vi "Trajectory_RelativeTo.vi"(9 "POSE":T3={"TRANSLATION"={"X"=0.0, "Y"=0.0}, "ROTATION"={"VALUE"=0.0, "COS"=1.0, "SIN"=0.0}} {"ROTATION"."SIN" format="%13.4f"; "ROTATION"."COS" format="%13.4f"; "ROTATION"."VALUE" format="%13.4f"; "TRANSLATION"."Y" format="%14.3f"; "TRANSLATION"."X" format="%14.3f"}, 11 "InputTRAJECTORY":T1 {"States"."POSE"."ROTATION"."SIN" format="%13.4f"; "States"."POSE"."ROTATION"."COS" format="%13.4f"; "States"."POSE"."ROTATION"."VALUE" format="%13.4f"; "States"."POSE"."TRANSLATION"."Y" format="%14.3f"; "States"."POSE"."TRANSLATION"."X" format="%14.3f"; "TotalTImeSecs" format="%20.3f"}) -> (3 "outputTRAJECTORY":T1 {"States"."POSE"."ROTATION"."SIN" format="%13.4f"; "States"."POSE"."ROTATION"."COS" format="%13.4f"; "States"."POSE"."ROTATION"."VALUE" format="%13.4f"; "States"."POSE"."TRANSLATION"."Y" format="%14.3f"; "States"."POSE"."TRANSLATION"."X" format="%14.3f"; "TotalTImeSecs" format="%20.3f"})   [LabVIEW 2019, in "Trajectory_Library.lvlib"]
doc: "Transforms all poses in the trajectory so that they are relative to the given pose. This is useful for converting a field-relative trajectory into a robot-relative trajectory.\n \nParameters:\n - InputTrajectory - Trajectory data structure\n - pose -The pose that is the origin of the coordinate frame that the current trajectory will be transformed into.\n \nReturns:\n - OutputTrajectory - The transformed trajectory."
uses:
  Trajectory_Library.lvlib
  TypeDef/TRANSLATION2D.ctl
  TypeDef/ROTATION2D.ctl
  TypeDef/POSE2D.ctl
  TypeDef/TRAJ_STATE.ctl
  TypeDef/TRAJECTORY.ctl
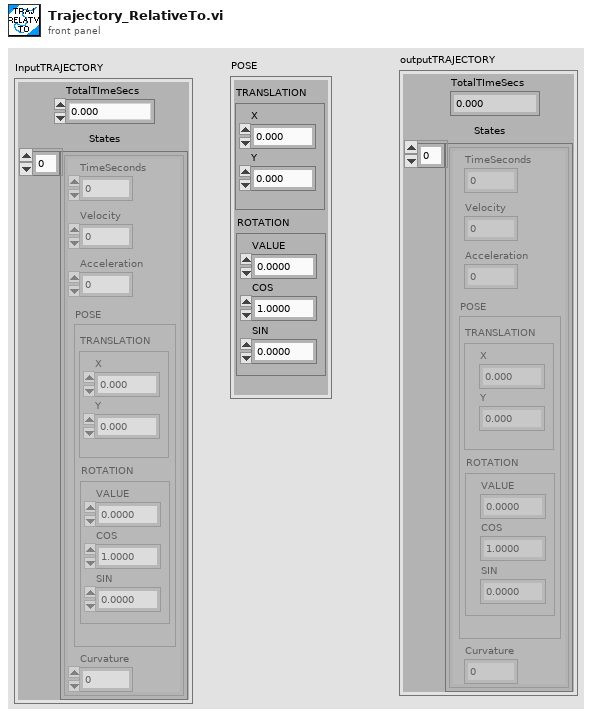
[diagram p1: front panel]
types:
  T1 = typedef "Trajectory_Library.lvlib/TRAJECTORY.ctl" = cluster{"TotalTImeSecs":dbl, "States":T2[]}
  T2 = typedef "Trajectory_Library.lvlib/TRAJ_STATE.ctl" = cluster{"TimeSeconds":dbl, "Velocity":dbl, "Acceleration":dbl, "POSE":T3, "Curvature":dbl}
  T3 = typedef "Trajectory_Library.lvlib/POSE2D.ctl" = cluster{"TRANSLATION":T4, "ROTATION":T5}
  T4 = typedef "Trajectory_Library.lvlib/TRANSLATION2D.ctl" = cluster{"X":dbl, "Y":dbl}
  T5 = typedef "Trajectory_Library.lvlib/ROTATION2D.ctl" = cluster{"VALUE":dbl, "COS":dbl, "SIN":dbl}
  T6 = typedef "WPILib_Math.lvlib/TRAJ_STATE.ctl" = cluster{"TimeSeconds":dbl, "Velocity":dbl, "Acceleration":dbl, "POSE":T7, "Curvature":dbl}
  T7 = typedef "WPILib_Math.lvlib/POSE2D.ctl" = cluster{"TRANSLATION":T8, "ROTATION":T9}
  T8 = typedef "WPILib_Math.lvlib/TRANSLATION2D.ctl" = cluster{"X":dbl, "Y":dbl}
  T9 = typedef "WPILib_Math.lvlib/ROTATION2D.ctl" = cluster{"VALUE":dbl, "COS":dbl, "SIN":dbl}
  T10 = typedef "WPILib_Math.lvlib/TRAJECTORY.ctl" = cluster{"TotalTImeSecs":dbl, "States":T6[]}
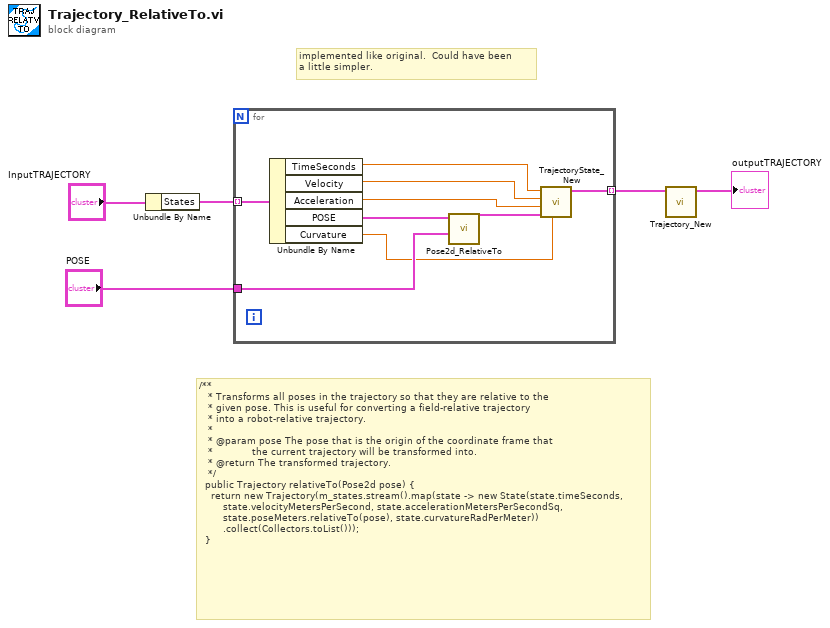
[diagram p0: block diagram]
diagram:
  # "implemented like original.  Could have been \na little simpler."
  # "/**\n   * Transforms all poses in the trajectory so that they are relative to the\n   * given pose. This is useful for converting a field-relative trajectory\n   * into a robot-relative trajectory.\n   *\n   * @param pose The pose that is the origin of the coordinate frame that\n   *             the current trajectory will be transformed into.\n   * @return The transformed trajectory.\n   */\n  public Trajectory relativeTo(Pose2d pose) {\n    return new Trajectory(m_states.stream().map(state -> new State(state.timeSeconds,\n        state.velocityMetersPerSecond, state.accelerationMetersPerSecondSq,\n        state.poseMeters.relativeTo(pose), state.curvatureRadPerMeter))\n        .collect(Collectors.toList()));\n  }"
  n1 = Unbundle By Name("InputTRAJECTORY") -> ("States"=w4:T2[])
  n2 = for {
    tunnel: w4 -> [w13] mode=indexing
    tunnel: [w14] -> w2 mode=indexing
    tunnel: "POSE" -> [w11]
    n3 = Unbundle By Name(w13) -> ("TimeSeconds"=w10:dbl, "Velocity"=w9:dbl, "Acceleration"=w8:dbl, "POSE"=w12:T3, "Curvature"=w6:dbl)
    n4 = call "Pose2d_RelativeTo.vi"("other POSE"=w11, "in POSE"=w12) -> ("out POSE"=w7:T3)  [unwired: 9 in]
    n5 = call "TrajectoryState_New.vi"("Curvature"=w6, "POSE"=w7, "Accel"=w8, "Velocity"=w9, "Time"=w10) -> ("TRAJ_STATE"=w14:T6)  [unwired: 6 in]
  }
  n6 = call "Trajectory_New.vi"("TRAJ_STATES"=w2) -> ("TRAJECTORY"=→"outputTRAJECTORY":T10)  [unwired: 10 in]
